vi "Main.vi"() -> ()   [LabVIEW 2019]
uses:
  <vilib>/sound2/lvsound2.llb/Sound Data Format.ctl
  <vilib>/sound2/lvsound2.llb/Sampling Mode.ctl
  <vilib>/sound2/lvsound2.llb/Sound File Refnum.ctl
  <vilib>/sound2/lvsound2.llb/Sound Input Read (DBL).vi
panel:
  out "Raw Data":waveform(dbl)[](graph)
  out "Spectrum Data":cluster{"f0":dbl, "df":dbl, "magnitude":dbl[]}[](graph)
  out "Threshold Exceeded?":bool
  in  "Threshold, dB":dbl=-100.0 format="%#_13g"
  in  "Upper Fc":dbl=3500.0 format="%#_13g"
  in  "Lower Fc":dbl=300.0 format="%#_13g"
  in  "Order":i32=6
  in  "Type":T1(ring)
  in  "Stop":bool
  # "FILTER SETTINGS"
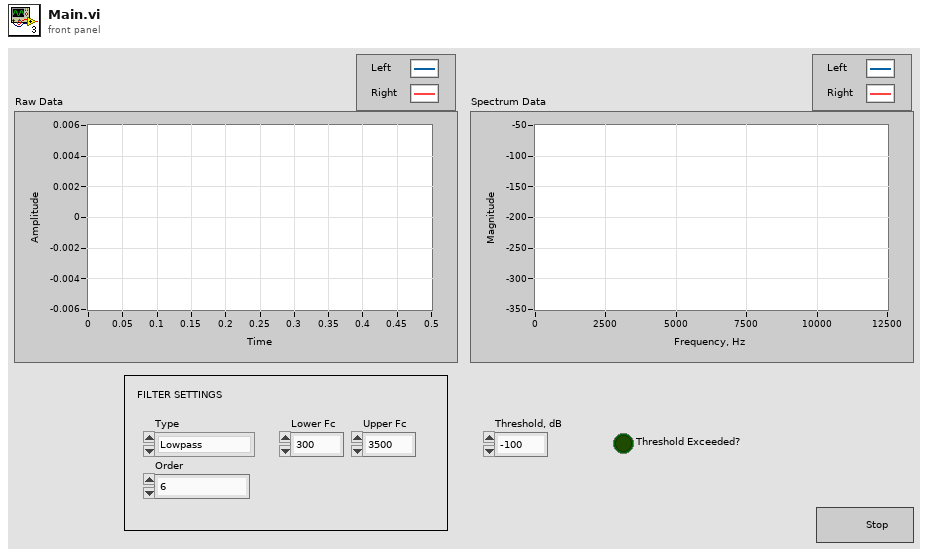
[diagram p1: front panel]
types:
  T1 = enum16{"Lowpass", "Highpass", "Bandpass", "Bandstop"}
  T2 = typedef "Sound File Refnum.ctl" = refnum<file>
  T3 = typedef "Sampling Mode.ctl" = i32
  T4 = typedef "Sound Data Format.ctl" = cluster{"sample rate (S/s)":dbl, "number of channels":i32, "bits per sample":i32}
  T5 = typedef "Sound Input Task ID.ctl" = u32
  T6 = cluster{"Topology":enum16{"Off", "Butterworth", "Chebyshev", "Inverse Chebyshev", "Elliptic", "Bessel"}, "Type":enum16{"Lowpass", "Highpass", "Bandpass", "Bandstop"}, "Order":i32, "Lower Fc":dbl, "Upper Fc":dbl, "PB Ripple":dbl, "SB Attenuation":dbl}
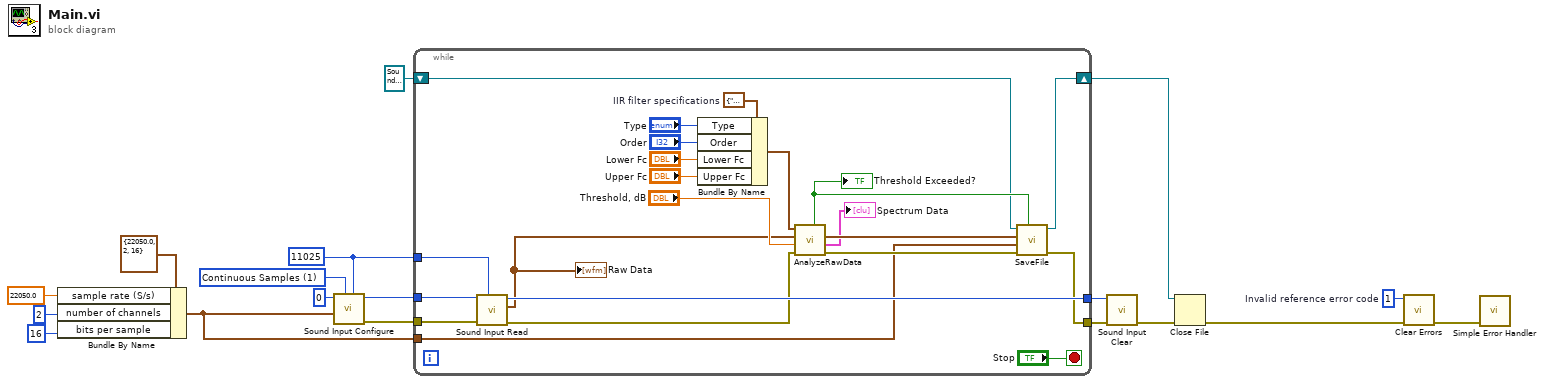
[diagram p0: block diagram]
diagram:
  w1 = 1  # Invalid reference error code
  w6 = 11025 ("Number of Samples/ch")
  w12 = T3 1 items=["Finite Samples", "Continuous Samples"] ("sample mode")
  n1 = Bundle By Name(cluster=T4 {"sample rate (S/s)"=22050.0, "number of channels"=2, "bits per sample"=16} ("sound format"), "sample rate (S/s)"=22050.0 ("Sample rate (Hz)"), "number of channels"=2 ("#Channels"), "bits per sample"=16 ("Resolution (bits)")) -> (w10:T4)
  n2 = call <vilib>:"Sound Input Configure.vi"("number of samples/ch"=w6, "sample mode"=w12, "sound format"=w10, "device ID"=u32 0 ("Device")) -> ("error out"=w18:errorcluster, "task ID"=w11:T5)  [unwired: 6 in]
  n3 = while {
    tunnel: w18 -> [w40]
    tunnel: w11 -> [w39]
    tunnel: w6 -> [w38]
    tunnel: w10 -> [w22]
    tunnel: [w23] -> w9
    tunnel: [w32] -> w7
    shift-right: [w20] -> w3
    shift-left: T2 refnum ("sound file refnum out") -> [w19]
    stop <- "Stop" stop-if-true
    w37 = T6 {"Topology"=enum."Butterworth", "Type"=enum."Lowpass", "Order"=1, "Lower Fc"=100.0, "Upper Fc"=200.0, "PB Ripple"=1.0, "SB Attenuation"=60.0}  # IIR filter specifications
    n4 = call-poly <vilib>:"Sound Input Read.vi"("number of samples/ch"=w38, "error in (no error)"=w40, "task ID"=w39) -> ("error out"=w30:errorcluster, "data"=w28:waveform(dbl)[], "task ID out"=w32:T5)  [unwired: 6 in]
    "Raw Data" <- w28
    n5 = Bundle By Name(cluster=w37, "Type"="Type", "Order"="Order", "Lower Fc"="Lower Fc", "Upper Fc"="Upper Fc") -> (w27:T6)
    n6 = call "AnalyzeRawData.vi"("error in (no error)"=w30, "Threshold, dB"="Threshold, dB", "Raw Data"=w28, "IIR Filter Specifications"=w27) -> ("error out"=w24:errorcluster, "Power Spectrum / PSD"=→"Spectrum Data":cluster{"f0":dbl, "df":dbl, "magnitude":dbl[]}[], "Filtered Data"=w26:waveform(dbl)[], "Threshold Exceeded?"=w21:bool)  [unwired: 4 in]
    "Threshold Exceeded?" <- w21
    n7 = call "SaveFile.vi"("Threshold Exceeded?"=w21, "error in (no error)"=w24, "sound format"=w22, "Filtered Data"=w26, "sound file refnum in"=w19) -> ("error out"=w23:errorcluster, "sound file refnum out"=w20:T2)  [unwired: 5 in]
  }
  n8 = call <vilib>:"Sound Input Clear.vi"("error in (no error)"=w9, "task ID"=w7) -> ("error out"=w8:errorcluster)  [unwired: 9 in]
  n9 = Close File(refnum=w3, error in=w8) -> (error out=w4:errorcluster)  [unwired: 1 out]
  n10 = call <vilib>:"Clear Errors.vi"("error in (no error)"=w4, "specific error code to clear (0: all)"=w1) -> ("error out"=w2:errorcluster)  [unwired: 4 in, 1 out]
  n11 = call <vilib>:"Simple Error Handler.vi"("error in (no error)"=w2) -> ()  [unwired: 4 in, 5 out]
